vi "Get N spatial streams.vi"(8 "error in (no error)":errorcluster, 11 "niDTS WLAN Dut Data in":refnum<class "niDTS WLAN Dut Data.lvclass">) -> (0 "error out":errorcluster, 2 "N spatial streams":cluster{"Value":i32, "Init":bool}={"Value"=1, "Init"=FALSE}, 3 "niDTS WLAN Dut Data out":refnum<class "niDTS WLAN Dut Data.lvclass">)   [LabVIEW 2015, in "niDTS WLAN.lvlib" / "niDTS WLAN Dut Data.lvclass"]
uses:
  niDTS WLAN Dut Data.lvclass
  niDTS WLAN Dut Data.lvclass/niDTS WLAN Dut Data.ctl
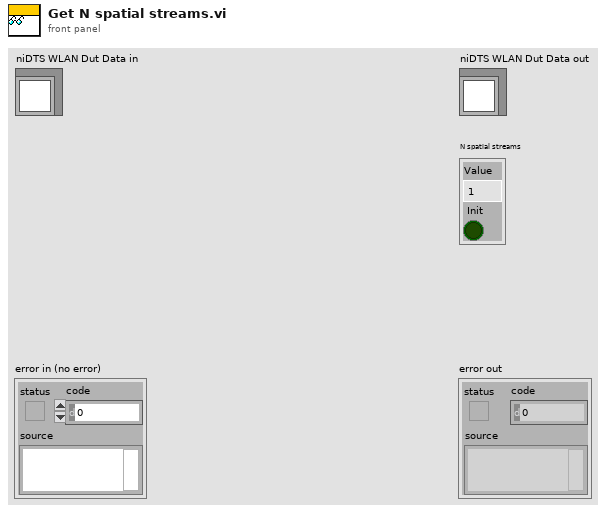
[diagram p1: front panel]
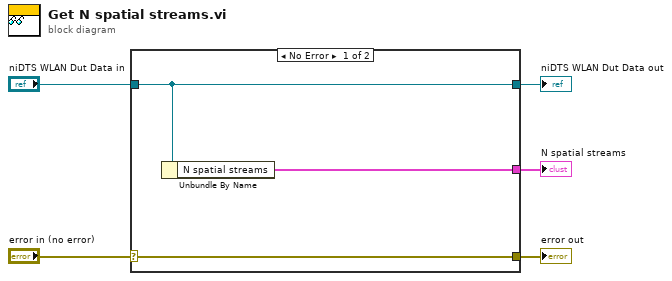
[diagram p0: block diagram]
diagram:
  n1 = case shown="No Error" "error in (no error)" {
    selector: "error in (no error)" -> [w8 w9]
    tunnel: [w8 w9] -> w4
    tunnel: [w7 w10] -> w2
    tunnel: "niDTS WLAN Dut Data in" -> [w7 w10]
    tunnel: [w6 _] -> w1
    frame No Error {
      n2 = Unbundle By Name(w7) -> ("N spatial streams"=w6:cluster{"Value":i32, "Init":bool})
    }
    frame Error {
    }
  }
  "error out" <- w4
  "niDTS WLAN Dut Data out" <- w2
  "N spatial streams" <- w1
